vi "SECADO_JKI.vi"() -> ()   [LabVIEW 2017] (continued)
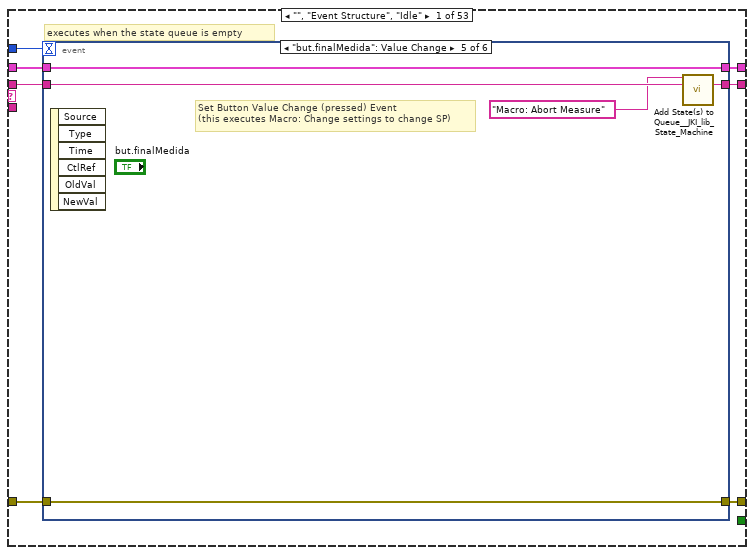
[diagram p2: hidden frame]
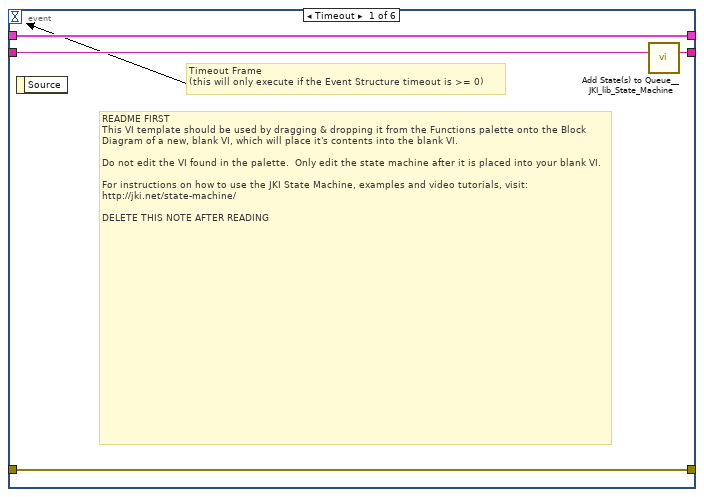
[diagram p3: hidden frame]
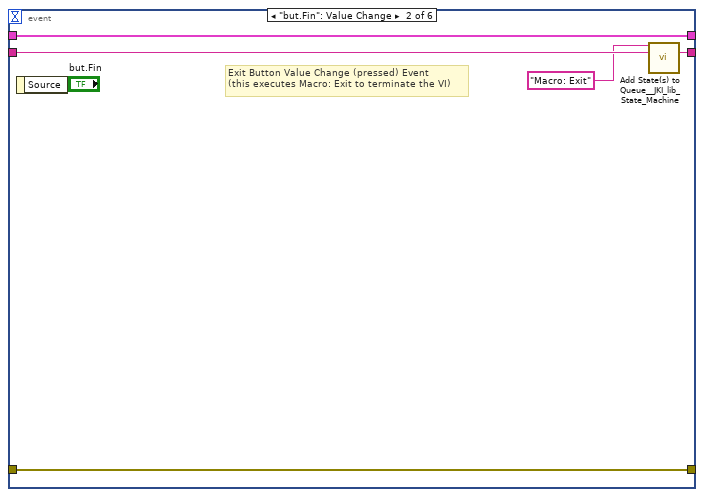
[diagram p4: hidden frame]
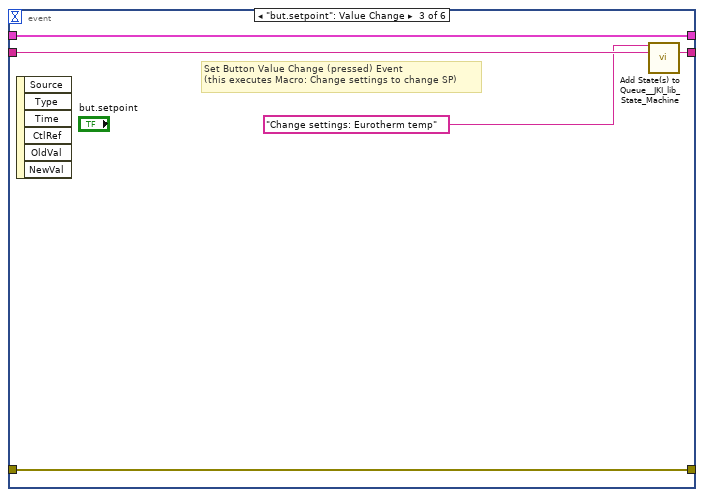
[diagram p5: hidden frame]
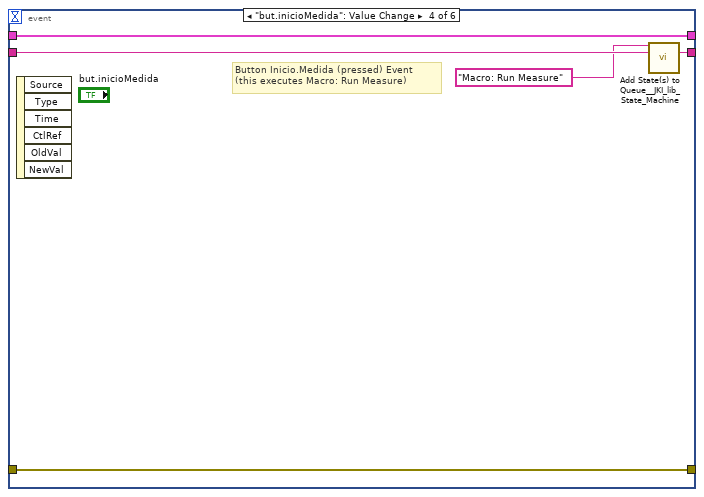
[diagram p6: hidden frame]
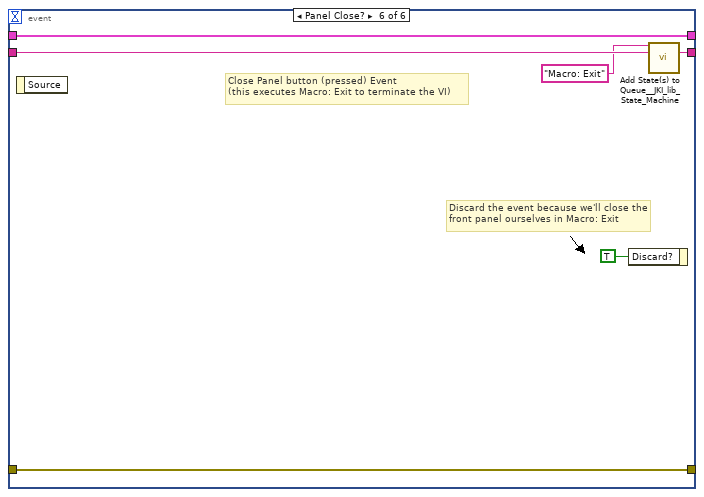
[diagram p7: hidden frame]
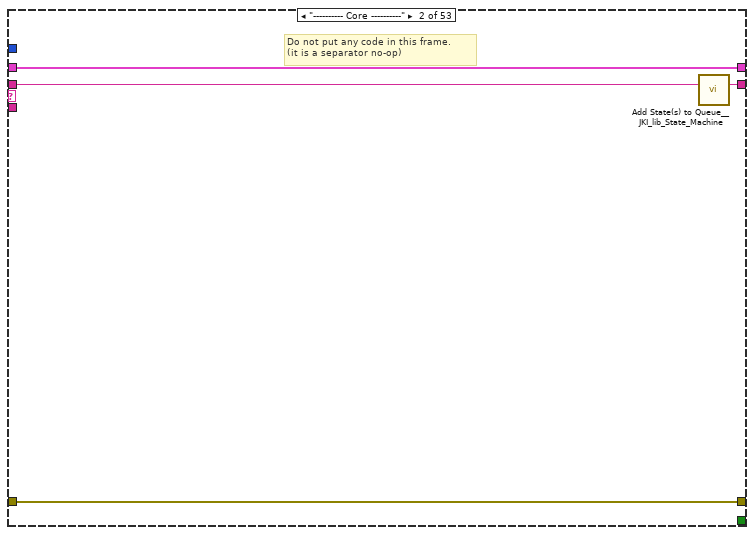
[diagram p8: hidden frame]
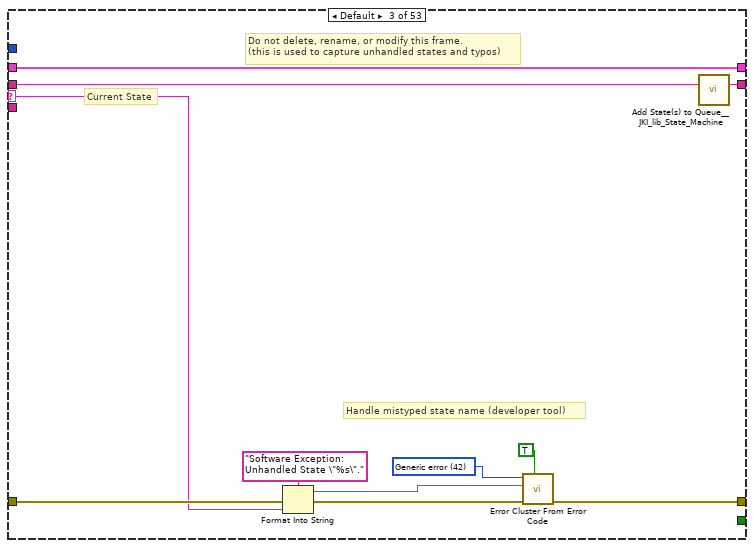
[diagram p9: hidden frame]
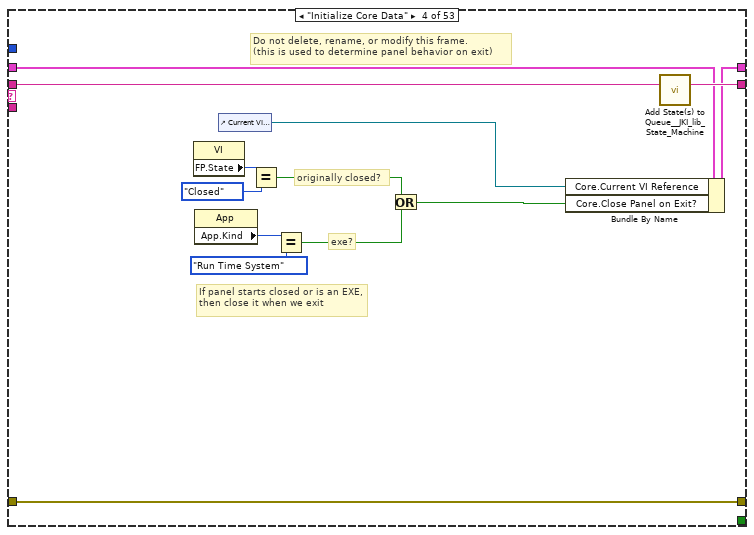
[diagram p10: hidden frame]
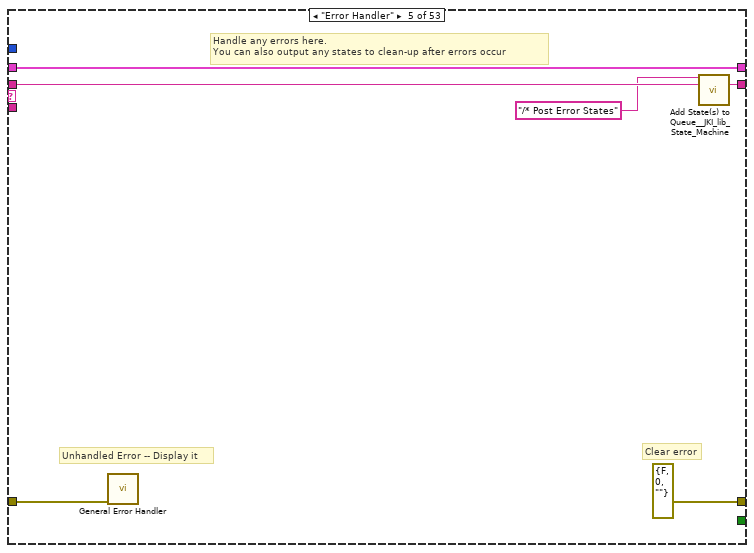
[diagram p11: hidden frame]
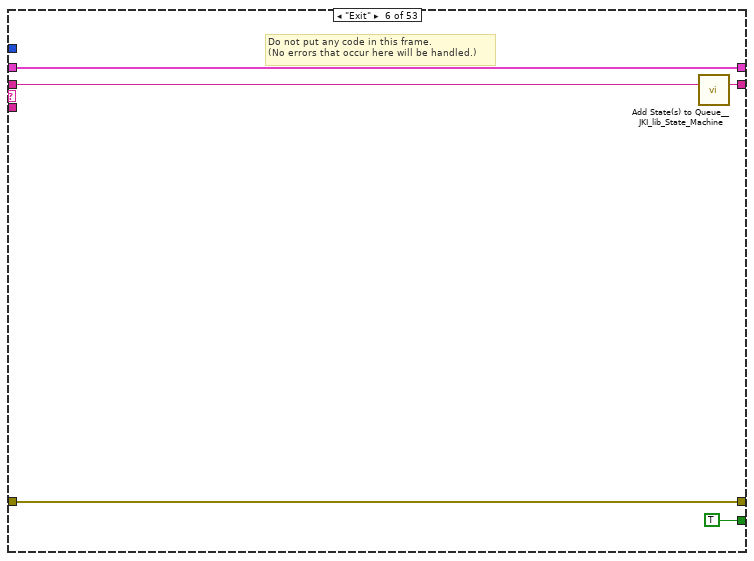
[diagram p12: hidden frame]
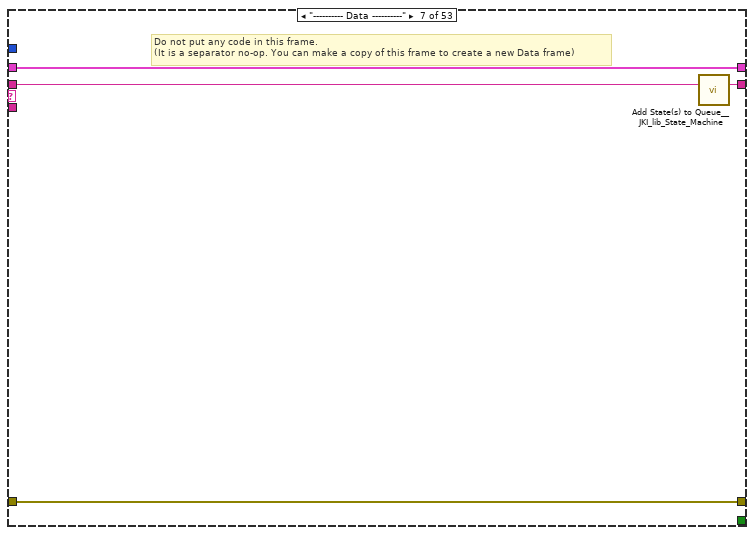
[diagram p13: hidden frame]
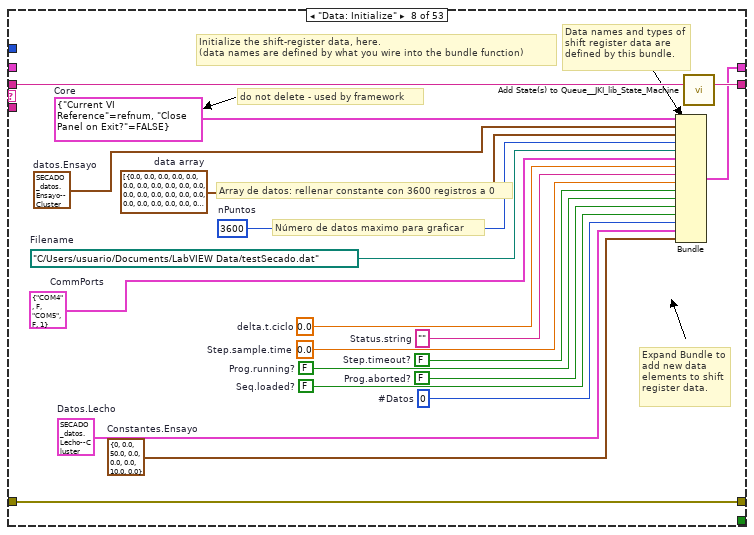
[diagram p14: hidden frame]
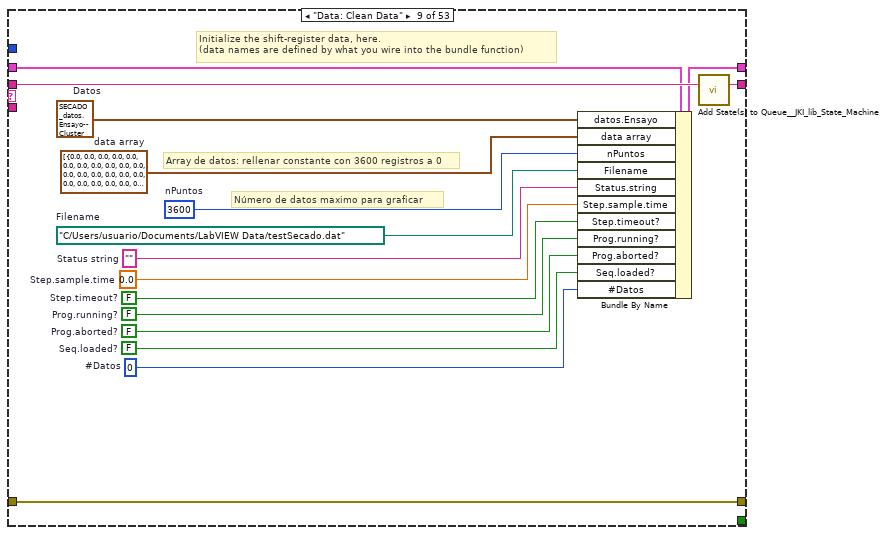
[diagram p15: hidden frame]
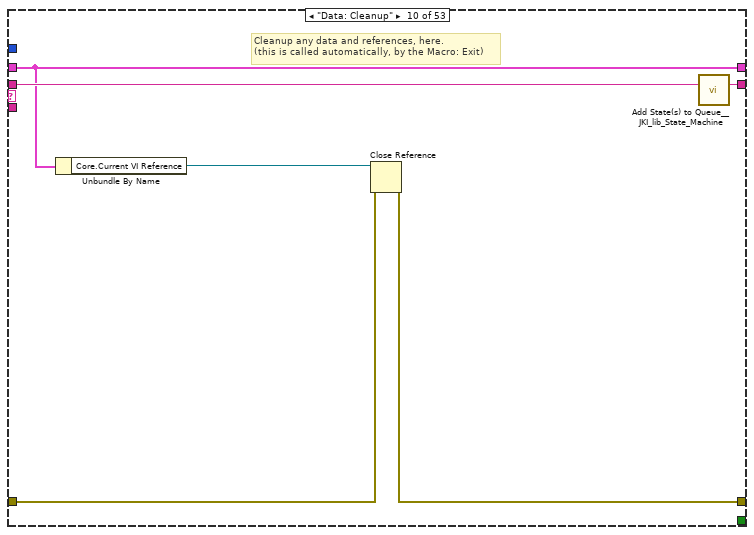
[diagram p16: hidden frame]
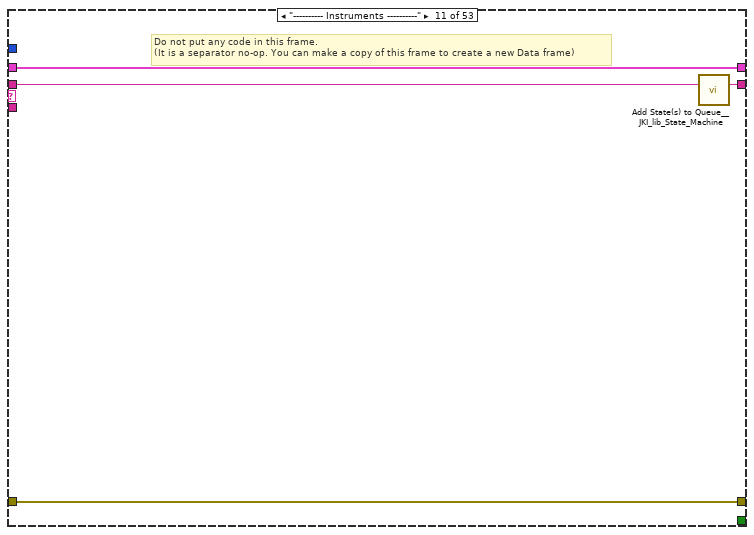
[diagram p17: hidden frame]
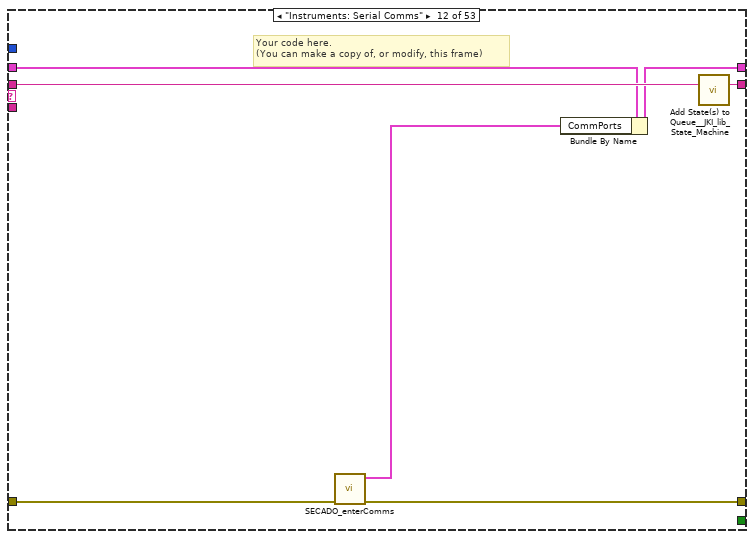
[diagram p18: hidden frame]
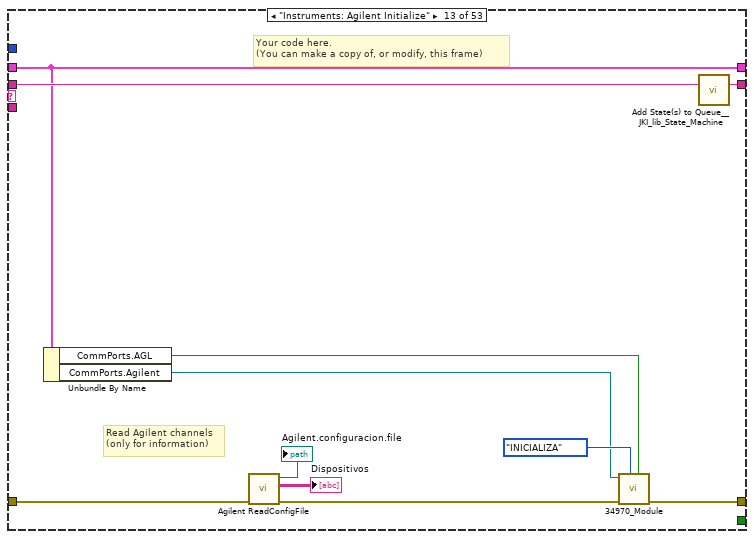
[diagram p19: hidden frame]
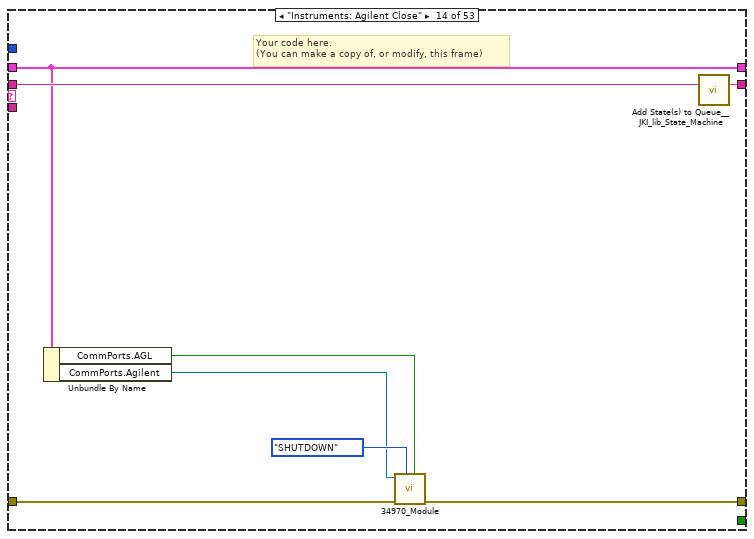
[diagram p20: hidden frame]
          tunnel: [w438] -> w406 mode=indexing
          tunnel: [w437] -> w407 mode=indexing
          tunnel: [w436] -> w408 mode=indexing
          tunnel: [w435] -> w409 mode=indexing
          tunnel: [w434] -> w410 mode=indexing
          tunnel: [w433] -> w399 mode=indexing
          tunnel: [w432] -> w400 mode=indexing
          tunnel: [w431] -> w401 mode=indexing
          tunnel: [w430] -> w402 mode=indexing
          tunnel: [w429] -> w403 mode=indexing
          tunnel: w396 -> [w428] mode=indexing
          tunnel: [w427] -> w371 mode=indexing
          tunnel: [w426] -> w370 mode=indexing
          tunnel: [w425] -> w369 mode=indexing
          tunnel: [w424] -> w368 mode=indexing
          tunnel: [w423] -> w367 mode=indexing
          tunnel: [w422] -> w366 mode=indexing
          tunnel: [w421] -> w365 mode=indexing
          tunnel: [w420] -> w364 mode=indexing
          tunnel: [w419] -> w363 mode=indexing
          tunnel: [w418] -> w351 mode=indexing
          n120 = Unbundle By Name(w428) -> ("Tiempo (min)"=w441:dbl, "P116.set.temp, C"=w440:dbl, "P116.temperatura, C"=w439:dbl, "Temp.pt100.1, C"=w438:dbl, "Temp.pt100.2, C"=w437:dbl, "Q.set.caudal, g/s"=w436:dbl, "Q.caudal, g/s"=w435:dbl, "P116.output, W"=w434:dbl, "Humedad.lecho, f1"=w433:dbl, "Agua.evapor, g/s"=w432:dbl, "Q.aire.seco, W"=w431:dbl, "Q.evaporacion, W"=w430:dbl, "Temperatura.ext, C"=w429:dbl, "Temp.pt100.3, C"=w427:dbl, "Temp.pt100.4, C"=w426:dbl, "Temp.termopar.5, C"=w425:dbl, "Temp.termopar.6, C"=w424:dbl, "Humedad.rel.3, f1"=w423:dbl, "Humedad.rel.4, f1"=w422:dbl, "Presion.dif, Pa"=w421:dbl, "Vel.arrastre, m/s"=w420:dbl, "Vel.arrastre, m/s"=w419:dbl, "Vel.arrastre, m/s"=w418:dbl)
        }
        n121 = Bundle(w352, w404) -> (w394:cluster{dbl[], dbl[]})  [unwired: 1 in]
        n122 = Bundle(w352, w405) -> (w393:cluster{dbl[], dbl[]})  [unwired: 1 in]
        n123 = Bundle(w352, w406) -> (w392:cluster{dbl[], dbl[]})  [unwired: 1 in]
        n124 = Bundle(w352, w407) -> (w391:cluster{dbl[], dbl[]})  [unwired: 1 in]
        n125 = Bundle(w352, w408) -> (w390:cluster{dbl[], dbl[]})  [unwired: 1 in]
        n126 = Bundle(w352, w409) -> (w389:cluster{dbl[], dbl[]})  [unwired: 1 in]
        n127 = Bundle(w352, w410) -> (w388:cluster{dbl[], dbl[]})  [unwired: 1 in]
        n128 = Bundle(w352, w399) -> (w387:cluster{dbl[], dbl[]})  [unwired: 1 in]
        n129 = Bundle(w352, w400) -> (w386:cluster{dbl[], dbl[]})  [unwired: 1 in]
        n130 = Bundle(w352, w401) -> (w385:cluster{dbl[], dbl[]})  [unwired: 1 in]
        n131 = Bundle(w352, w402) -> (w384:cluster{dbl[], dbl[]})  [unwired: 1 in]
        n132 = Bundle(w352, w403) -> (w377:cluster{dbl[], dbl[]})  [unwired: 1 in]
        n133 = Bundle(w352, w371) -> (w362:cluster{dbl[], dbl[]})  [unwired: 1 in]
        n134 = Bundle(w352, w370) -> (w361:cluster{dbl[], dbl[]})  [unwired: 1 in]
        n135 = Bundle(w352, w369) -> (w360:cluster{dbl[], dbl[]})  [unwired: 1 in]
        n136 = Bundle(w352, w368) -> (w359:cluster{dbl[], dbl[]})  [unwired: 1 in]
        n137 = Bundle(w352, w367) -> (w358:cluster{dbl[], dbl[]})  [unwired: 1 in]
        n138 = Bundle(w352, w366) -> (w357:cluster{dbl[], dbl[]})  [unwired: 1 in]
        n139 = Bundle(w352, w365) -> (w356:cluster{dbl[], dbl[]})  [unwired: 1 in]
        n140 = Bundle(w352, w364) -> (w355:cluster{dbl[], dbl[]})  [unwired: 1 in]
        n141 = Bundle(w352, w363) -> (w354:cluster{dbl[], dbl[]})  [unwired: 1 in]
        n142 = Bundle(w352, w351) -> (w353:cluster{dbl[], dbl[]})  [unwired: 1 in]
        n143 = Build Array(w387) -> (→"CONCENTRACION HUMEDAD":cluster{dbl[], dbl[]}[])
        n144 = Build Array(w386) -> (→"AGUA EVAPORADA AL AIRE":cluster{dbl[], dbl[]}[])
        n145 = Build Array(w394, w393, w392, w391) -> (→"EUROTHERM":cluster{dbl[], dbl[]}[])
        n146 = Build Array(w390, w389) -> (→"CAUDAL":cluster{dbl[], dbl[]}[])
        n147 = Build Array(w388) -> (→"POTENCIA CALEFACCION":cluster{dbl[], dbl[]}[])
        n148 = Build Array(w385, w384) -> (→"Q CEDIDO Y ABSORBIDO":cluster{dbl[], dbl[]}[])
        n149 = Build Array(w358, w357) -> (→"HUMEDAD":cluster{dbl[], dbl[]}[])
        n150 = Build Array(w356) -> (→"PRES_DIF":cluster{dbl[], dbl[]}[])
        n151 = Build Array(w377, w362, w361, w360, w359) -> (→"TEMPERATURA":cluster{dbl[], dbl[]}[])
        n152 = Build Array(w355, w354, w353) -> (→"VELOCIDADES":cluster{dbl[], dbl[]}[])
        n153 = Bundle By Name(cluster=w415, "data array"=w396) -> (w397:T18)
        n154 = call <vilib>:"Add State(s) to Queue__JKI_lib_State_Machine.vi"("State(s) in (\"\")"=w417) -> ("States Out"=w416:string)  [unwired: 14 in]
      }
      frame "---------- Macro ----------" {
        # "Do not put any code in this frame.\n(It is a separator no-op. You can make a copy of this frame to create a new Macro frame)"
        n155 = call <vilib>:"Add State(s) to Queue__JKI_lib_State_Machine.vi"("State(s) in (\"\")"=w445) -> ("States Out"=w444:string)  [unwired: 14 in]
      }
      frame "Macro: Inicializar" {
        w452 = "Data: Initialize\nData: Clean Data\nInitialize Core Data\nUI: Initialize\nUI: Front Panel State >> Open\nMacro: Interlock\nUI: Update Meas Data\nUI: Update Graphics\nInstruments: Serial Comms\nInstruments: Agilent Initialize\nInstruments: Eurotherm Initialize"  # Data: Initialize Data: Clean Data Initialize Core Data UI: Initialize UI: Front Panel State >> Open Macro: Interlock UI: Update Meas Data UI: Update Graphics Instruments: Serial Comms Instruments: Agilent Initialize Instruments: Eurotherm Initialize
        # "Initialization Macro\n(This is called once, when the VI starts)"
        n156 = Bundle By Name(cluster=w447, "Prog.running?"=TRUE ("Prog. Running?"), "Prog.aborted?"=FALSE ("Prog. Aborted?"), "Seq.loaded?"=FALSE ("Seq. Loaded?"), "Status.string"="Ready to start...") -> (w446:T18)
        n157 = call <vilib>:"Add State(s) to Queue__JKI_lib_State_Machine.vi"("State(s) in Front (\"\")"=w452, "State(s) in (\"\")"=w455) -> ("States Out"=w454:string)  [unwired: 13 in]
      }
      frame "Macro: Run Measure" {
        # "Run Measure Macro\n(This is called once, when the VI starts)"
        n158 = Bundle By Name(cluster=w462, "Prog.running?"=TRUE ("Prog. Running?"), "Prog.aborted?"=FALSE ("Prog. Aborted?"), "Seq.loaded?"=FALSE ("Seq. Loaded?"), "Status.string"="Adquisition in progress...") -> (w460:T18)
        n159 = call <vilib>:"Add State(s) to Queue__JKI_lib_State_Machine.vi"("State(s) in Front (\"\")"="UI: Initialize\nMacro: Interlock\nFile: Filename\nTiming: Initialize Total Time\nTiming: Initialize Sample Time\nMacro: Next Meas Cycle", "State(s) in (\"\")"=w465) -> ("States Out"=w464:string)  [unwired: 13 in]
      }
      frame "Macro: Abort Measure" {
        # "Abort Measure Macro\n(This is called when abort buton is pressed)"
        n160 = Bundle By Name(cluster=w470, "Prog.running?"=FALSE ("Prog. Running?"), "Prog.aborted?"=TRUE ("Prog. Aborted?"), "Seq.loaded?"=FALSE ("Seq. Loaded?"), "Status.string"="Adquisition aborted...") -> (w469:T18)
        n161 = One Button Dialog(message="Measure aborted") -> ()  [unwired: 1 in, 1 out]
        n162 = call <vilib>:"Add State(s) to Queue__JKI_lib_State_Machine.vi"("State(s) in (\"\")"="// Data: Set Seq. Aborted Flag >> True\n// Macro: Interlock\n// IO: Dwell  // finish current step (remove to abort immediately)\n// Data: Set Running Step >> -1\n// UI: Update Table Selection\n// Data: Set Seq. Aborted Flag >> False\nMacro: Interlock") -> ("States Out"=w475:string)  [unwired: 14 in]
      }
      frame "Macro: Next Meas Cycle" {
        # "Initialization Macro\n(This is called once, when the VI starts)"
        n163 = Unbundle By Name(w479) -> ("#Datos"=w477:i32)
        n164 = Increment(x=w477) -> (x+1=w476:i32)
        "#.datos" <- w476
        n165 = Bundle By Name(cluster=w479, "#Datos"=w476) -> (w478:T18)
        n166 = call <vilib>:"Add State(s) to Queue__JKI_lib_State_Machine.vi"("State(s) in Front (\"\")"="Timing: Measure Total Time\nMacro: Take Data\nMacro: Calculate\nMacro: Interlock\nFile: Save Data\nUI: Update Meas Data\nUI: Update Graphics\nSampling: Check For Next Sample", "State(s) in (\"\")"=w483) -> ("States Out"=w482:string)  [unwired: 13 in]
      }
      frame "Macro: Take Data" {
        # "Initialization Macro\n(This is called once, when the VI starts)"
        n167 = call <vilib>:"Add State(s) to Queue__JKI_lib_State_Machine.vi"("State(s) in Front (\"\")"="Measure data: Agilent Temp.PT100\nMeasure data: Agilent Temp.TERMOPAR\nMeasure data: Agilent Pressure\nMeasure data: Agilent Humidity\nMeasure data: Eurotherm Temperature", "State(s) in (\"\")"=w488) -> ("States Out"=w487:string)  [unwired: 13 in]
      }
      frame "Macro: Calculate" {
        # "Initialization Macro\n(This is called once, when the VI starts)"
        n168 = call <vilib>:"Add State(s) to Queue__JKI_lib_State_Machine.vi"("State(s) in Front (\"\")"="Calculations: Calculos 1", "State(s) in (\"\")"=w493) -> ("States Out"=w492:string)  [unwired: 13 in]
      }
      frame "Macro: Interlock" {
        # "Initialization Macro\n(This is called once, when the VI starts)"
        n169 = call <vilib>:"Add State(s) to Queue__JKI_lib_State_Machine.vi"("State(s) in Front (\"\")"="UI: Update Status\nUI: Update Interlock", "State(s) in (\"\")"=w498) -> ("States Out"=w497:string)  [unwired: 13 in]
      }
      frame "Macro: Exit" {
        # "Exit Macro\n(This is called once, when the VI exits)"
        n170 = Unbundle By Name(w506) -> ("Core.Close Panel on Exit?"=w505:bool)
        n171 = One Button Dialog(message="Program stop") -> ()  [unwired: 1 in, 1 out]
        n172 = Select(t="UI: Front Panel State >> Close", s=w505, f="") -> (s? t:f=w502:string)
        n173 = call <vilib>:"Add State(s) to Queue__JKI_lib_State_Machine.vi"("State(s) in (\"\")"=w502, "State(s) at Back (\"\")"="Data: Cleanup\nExit") -> ("States Out"=w500:string)  [unwired: 13 in]
        n174 = call <vilib>:"Add State(s) to Queue__JKI_lib_State_Machine.vi"("State(s) in Front (\"\")"=w500, "State(s) in (\"\")"=w509) -> ("States Out"=w508:string)  [unwired: 13 in]
      }
      frame "---------- File ----------" {
        # "Template Separator\n(You can make a copy of, or modify, this frame)"
        n175 = call <vilib>:"Add State(s) to Queue__JKI_lib_State_Machine.vi"("State(s) in (\"\")"=w513) -> ("States Out"=w512:string)  [unwired: 14 in]
      }
      frame "File: Filename" {
        # "Al arrancar la medida:\nHumedad.lecho = Humedad_inicial"
        # "Initialize and save head data"
        # "Your code here.\n(You can make a copy of, or modify, this frame)"
        n176 = call "SECADO_enterEnsayo.vi"("error in (no error)"=w520) -> ("error out"=w522:errorcluster, "Datos.Lecho"=w515:T5, "Constantes.Ensayo"=w516:T6)  [unwired: 7 in, 1 out]
        "Constantes.Ensayo" <- w516
        "Datos.Lecho" <- w515
        n177 = Unbundle By Name(w515) -> ("Hum_ini, %"=w514:dbl)
        n178 = call "File_Module.vi"("Command"=File_Module_Control."Initialize", "error in (no error)"=w522, "Datos.Lecho"=w515, "Constantes.Ensayo"=w516) -> ("error out"=w519:errorcluster, "selected path"=w517:path)  [unwired: 6 in]
        "Fichero" <- w517
        n179 = Bundle By Name(cluster=w523, "Constantes.Ensayo"=w516, "Datos.Lecho"=w515, "Filename"=w517, "datos.Ensayo.Humedad.lecho, f1"=w514) -> (w518:T18)
        n180 = call <vilib>:"Add State(s) to Queue__JKI_lib_State_Machine.vi"("State(s) in (\"\")"=w525) -> ("States Out"=w524:string)  [unwired: 14 in]
      }
      frame "File: Save Data" {
        # "Your code here.\n(You can make a copy of, or modify, this frame)"
        n181 = Get Date/Time String() -> (date string=→"Fecha":string, time string=→"Hora":string)  [unwired: 3 in]
        n182 = Unbundle By Name(w528) -> ("datos.Ensayo"=w529:T4)
        n183 = call "File_Module.vi"("Command"=File_Module_Control."Save Data", "error in (no error)"=w531, "Datos.Ensayo"=w529) -> ("error out"=w530:errorcluster)  [unwired: 7 in, 1 out]
        n184 = call <vilib>:"Add State(s) to Queue__JKI_lib_State_Machine.vi"("State(s) in (\"\")"=w534) -> ("States Out"=w533:string)  [unwired: 14 in]
      }
      frame "---------- Sampling ----------" {
        # "Template Separator\n(You can make a copy of, or modify, this frame)"
        n185 = call <vilib>:"Add State(s) to Queue__JKI_lib_State_Machine.vi"("State(s) in (\"\")"=w538) -> ("States Out"=w537:string)  [unwired: 14 in]
      }
      frame "Sampling: Check For Next Sample" {
        # "Your code here.\n(You can make a copy of, or modify, this frame)"
        n186 = Unbundle By Name(w544) -> ("Step.timeout?"=w542:bool)
        n187 = Select(t="Timing: Initialize Sample Time\nMacro: Next Meas Cycle", s=w542, f="Idle  //Calls event structure\nTiming: Measure Sample Time\nSampling: Check For Next Sample // Come back here") -> (s? t:f=w540:string)
        n188 = call <vilib>:"Add State(s) to Queue__JKI_lib_State_Machine.vi"("State(s) in Front (\"\")"=w540, "State(s) in (\"\")"=w546) -> ("States Out"=w545:string)  [unwired: 13 in]
      }
      frame "---------- Measure data ----------" {
        # "Template Separator\n(You can make a copy of, or modify, this frame)"
        n189 = call <vilib>:"Add State(s) to Queue__JKI_lib_State_Machine.vi"("State(s) in (\"\")"=w550) -> ("States Out"=w549:string)  [unwired: 14 in]
      }
      frame "Measure data: Agilent Temp.PT100" {
        # "Agilent temperature readings code here.\n(You can make a copy of, or modify, this frame)"
        n190 = Unbundle By Name(w553) -> ("CommPorts.AGL"=w551:bool, "CommPorts.Agilent"=w552:refnum<visa-resource-name>)
        n191 = call "34970_Module.vi"("Agilent 34970A"=w551, "Command"=34970_Module_Control."LECTURA PT100", "error in (no error)"=w554, "VISA Agilent 34970A"=w552) -> ("error out"=w555:errorcluster, "TEMP.PT100"=w561:dbl[])  [unwired: 3 in, 3 out]
        n192 = Index Array(array=w561) -> (element #1=w559:dbl, element #2=w558:dbl, element #3=w557:dbl, element #4=w556:dbl)  [unwired: 4 in]
        n193 = Bundle By Name(cluster=w553, "datos.Ensayo.Temp.pt100.1, C"=w559, "datos.Ensayo.Temp.pt100.2, C"=w558, "datos.Ensayo.Temp.pt100.3, C"=w557, "datos.Ensayo.Temp.pt100.4, C"=w556) -> (w560:T18)
        n194 = call <vilib>:"Add State(s) to Queue__JKI_lib_State_Machine.vi"("State(s) in (\"\")"=w564) -> ("States Out"=w563:string)  [unwired: 14 in]
      }
      frame "Measure data: Agilent Temp.TERMOPAR" {
        # "Agilent temperature readings code here.\n(You can make a copy of, or modify, this frame)"
        n195 = Unbundle By Name(w567) -> ("CommPorts.AGL"=w565:bool, "CommPorts.Agilent"=w566:refnum<visa-resource-name>)
        n196 = call "34970_Module.vi"("Agilent 34970A"=w565, "Command"=34970_Module_Control."LECTURA TERMOPAR", "error in (no error)"=w568, "VISA Agilent 34970A"=w566) -> ("error out"=w569:errorcluster, "TEMP.PT100"=w574:dbl[])  [unwired: 3 in, 3 out]
        n197 = Index Array(array=w574) -> (element #1=w572:dbl, element #2=w571:dbl, element #3=w570:dbl)  [unwired: 3 in]
        n198 = Bundle By Name(cluster=w567, "datos.Ensayo.Temperatura.ext, C"=w572, "datos.Ensayo.Temp.termopar.5, C"=w571, "datos.Ensayo.Temp.termopar.6, C"=w570) -> (w573:T18)
        n199 = call <vilib>:"Add State(s) to Queue__JKI_lib_State_Machine.vi"("State(s) in (\"\")"=w577) -> ("States Out"=w576:string)  [unwired: 14 in]
      }
      frame "Measure data: Agilent Pressure" {
        # "Agilent pressure readings code here.\n(You can make a copy of, or modify, this frame)"
        n200 = Unbundle By Name(w582) -> ("CommPorts.AGL"=w580:bool, "CommPorts.Agilent"=w581:refnum<visa-resource-name>)
        n201 = call "34970_Module.vi"("Agilent 34970A"=w580, "Command"=34970_Module_Control."LECTURA PRESION", "error in (no error)"=w583, "VISA Agilent 34970A"=w581) -> ("error out"=w584:errorcluster, "PRESION"=w578:dbl[])  [unwired: 3 in, 3 out]
        n202 = Index Array(array=w578) -> (element=w585:dbl)  [unwired: 1 in]
        n203 = Bundle By Name(cluster=w582, "datos.Ensayo.Presion.dif, Pa"=w585) -> (w586:T18)
        n204 = call <vilib>:"Add State(s) to Queue__JKI_lib_State_Machine.vi"("State(s) in (\"\")"=w588) -> ("States Out"=w587:string)  [unwired: 14 in]
      }
      frame "Measure data: Agilent Humidity" {
        # "Agilent humidity readings code here.\n(You can make a copy of, or modify, this frame)"
        n205 = Unbundle By Name(w593) -> ("CommPorts.AGL"=w591:bool, "CommPorts.Agilent"=w592:refnum<visa-resource-name>)
        n206 = call "34970_Module.vi"("Agilent 34970A"=w591, "Command"=34970_Module_Control."LECTURA HUMEDAD", "error in (no error)"=w594, "VISA Agilent 34970A"=w592) -> ("error out"=w595:errorcluster, "HUMEDAD"=w589:dbl[])  [unwired: 3 in, 3 out]
        n207 = Index Array(array=w589) -> (element #1=w597:dbl, element #2=w596:dbl)  [unwired: 2 in]
        n208 = Bundle By Name(cluster=w593, "datos.Ensayo.Humedad.rel.3, f1"=w597, "datos.Ensayo.Humedad.rel.4, f1"=w596) -> (w598:T18)
        n209 = call <vilib>:"Add State(s) to Queue__JKI_lib_State_Machine.vi"("State(s) in (\"\")"=w600) -> ("States Out"=w599:string)  [unwired: 14 in]
      }
      frame "Measure data: Eurotherm Temperature" {
        # "POTENCIA MAXIMA"
        # "Your code here.\n(You can make a copy of, or modify, this frame)"
        n210 = Unbundle By Name(w624) -> ("CommPorts.CDT"=w618:bool, "CommPorts.Eurotherm"=w619:refnum<visa-resource-name>, "CommPorts.#Dec"=w604:u16)
        n211 = local read "Constantes.Ensayo"() -> (w603:T6)
        n212 = Unbundle By Name(w603) -> ("Voltaje_resist, vac"=w601:dbl, "Resistencia, ohm"=w602:dbl)
        n213 = call "Eurotherm_2023_Module.vi"("Eurotherm (T:Enable)"=w618, "Command"=Eurotherm_2023_Module."Initialize", "error in (no error)"=w623, "VISA resource name"=w619) -> ("error out"=w616:errorcluster)  [unwired: 5 in, 2 out]
        n214 = Square(x=w601) -> (x^2=w612:dbl)
        n215 = call "Eurotherm_2023_Module.vi"("Decimales"=w604, "Eurotherm (T:Enable)"=w618, "Command"=Eurotherm_2023_Module."Read data", "error in (no error)"=w616, "Address"=Address."Add 1", "VISA resource name"=w619) -> ("error out"=w615:errorcluster, "Eurotherm"=w614:T20)  [unwired: 3 in, 1 out]
        n216 = Divide(x=w612, y=w602) -> (x/y=w611:dbl)
        n217 = Unbundle By Name(w614) -> ("workingSP"=w608:dbl, "processVal"=w607:dbl, "workingOut"=w605:dbl)
        n218 = Multiply(x=w605, y=w611) -> (x*y=w610:dbl)
        n219 = Divide(x=w610, y=100.0) -> (x/y=w606:dbl)
        n220 = call "Eurotherm_2023_Module.vi"("Eurotherm (T:Enable)"=w618, "Command"=Eurotherm_2023_Module."Shutdown", "error in (no error)"=w615, "VISA resource name"=w619) -> ("error out"=w621:errorcluster)  [unwired: 5 in, 2 out]
        n221 = Bundle By Name(cluster=w624, "datos.Ensayo.P116.set.temp, C"=w608, "datos.Ensayo.P116.temperatura, C"=w607, "datos.Ensayo.P116.output, %"=w605, "datos.Ensayo.P116.output, W"=w606) -> (w620:T18)
        n222 = call <vilib>:"Add State(s) to Queue__JKI_lib_State_Machine.vi"("State(s) in (\"\")"=w627) -> ("States Out"=w626:string)  [unwired: 14 in]
      }
      frame "---------- Change settings ----------" {
        # "Template Separator\n(You can make a copy of, or modify, this frame)"
        n223 = call <vilib>:"Add State(s) to Queue__JKI_lib_State_Machine.vi"("State(s) in (\"\")"=w631) -> ("States Out"=w630:string)  [unwired: 14 in]
      }
      frame "Change settings: Eurotherm temp" {
        # "Your code here.\n(You can make a copy of, or modify, this frame)"
        n224 = Unbundle By Name(w641) -> ("datos.Ensayo.P116.set.temp, C"=w633:dbl, "CommPorts"=w638:T17, "CommPorts.CDT"=w640:bool, "CommPorts.Eurotherm"=w639:refnum<visa-resource-name>, "CommPorts.#Dec"=w637:u16)
        n225 = Bundle By Name(cluster=T15 {"TargetSP"={"Ch1"=0.0}, "WorkingSP"={"Ch1"=0.0}, "Temperatura"={"Ch1"=0.0}, "RateSP"={"Ch1"=0.0}, "Potencia"={"Ch1"=0.0}, "Potencia max"={"Ch1"=0.0}} ("P116x1ch"), "RateSP.Ch1"=0.0, "TargetSP.Ch1"=w633) -> (w635:T15)
        n226 = call "Eurotherm_2023_Module.vi"("Eurotherm (T:Enable)"=w640, "Command"=Eurotherm_2023_Module."Initialize", "error in (no error)"=w642, "VISA resource name"=w639) -> ("error out"=w646:errorcluster)  [unwired: 5 in, 2 out]
        n227 = call "P116x1ch_WriteManual.vi"("P116x1ch"=w635, "Decimales"=w637, "error in (no error)"=w646, "Comunicaciones"=w638) -> ("error out"=w645:errorcluster)  [unwired: 5 in, 2 out]
        n228 = call "Eurotherm_2023_Module.vi"("Eurotherm (T:Enable)"=w640, "Command"=Eurotherm_2023_Module."Shutdown", "error in (no error)"=w645, "VISA resource name"=w639) -> ("error out"=w636:errorcluster)  [unwired: 5 in, 2 out]
        n229 = call <vilib>:"Add State(s) to Queue__JKI_lib_State_Machine.vi"("State(s) in (\"\")"=w648) -> ("States Out"=w647:string)  [unwired: 14 in]
      }
      frame "---------- Calculations ----------" {
        # "Template Separator\n(You can make a copy of, or modify, this frame)"
        n230 = call <vilib>:"Add State(s) to Queue__JKI_lib_State_Machine.vi"("State(s) in (\"\")"=w652) -> ("States Out"=w651:string)  [unwired: 14 in]
      }
      frame "Calculations: Calculos 1" {
        w655 = T2 {"Agua.evap, g/s"=0.0, "Hum.lecho, %"=1.0, "Q.aire.seco, W"=50.0, "Q.evaporacion, W"=230.0, "Porosidad"=60.0, "Vel.a.lecho, m/s"=1.0, "Vel.min.fluido, m/s"=10.0, "Vel.arrastre, m/s"=5.0}  # Calculos.Ensayo
        # "Set Front Panel Open or Closed\n(Usage: \"UI: Front Panel State >> Open|Close\")"
        n231 = Unbundle By Name(w667) -> ("Datos.Lecho"=w664:T5, "Constantes.Ensayo"=w665:T6, "datos.Ensayo"=w666:T4)
        n232 = call "SECADO_calculos.vi"("error in (no error)"=w669, "datos.Ensayo.in"=w666, "Constantes.Ensayo"=w665, "Datos.Lecho"=w664) -> ("error out"=w668:errorcluster, "datos.Ensayo.out"=w654:T4)  [unwired: 6 in]
        n233 = Unbundle By Name(w654) -> ("Agua.evapor, g/s"=w656:dbl, "Humedad.lecho, f1"=w657:dbl, "Q.aire.seco, W"=w658:dbl, "Q.evaporacion, W"=w659:dbl, "Porosidad,"=w660:dbl, "Vel.a.lecho, m/s"=w661:dbl, "Vel.min.fluido, m/s"=w662:dbl, "Vel.arrastre, m/s"=w663:dbl)
        n234 = Bundle By Name(cluster=w655, "Agua.evap, g/s"=w656, "Hum.lecho, %"=w657, "Q.aire.seco, W"=w658, "Q.evaporacion, W"=w659, "Porosidad"=w660, "Vel.a.lecho, m/s"=w661, "Vel.min.fluido, m/s"=w662, "Vel.arrastre, m/s"=w663) -> (→"Calculos.Ensayo":T2)
        n235 = Bundle By Name(cluster=w667, "datos.Ensayo"=w654) -> (w670:T18)
        n236 = call <vilib>:"Add State(s) to Queue__JKI_lib_State_Machine.vi"("State(s) in (\"\")"=w672) -> ("States Out"=w671:string)  [unwired: 14 in]
      }
    }
    n237 = call <userlib>:"Wait (ms)__ogtk.vi"("error in (no error)"=w8, "milliseconds to wait"="t.wait, ms") -> ("error out"=w6:errorcluster)  [unwired: 8 in, 1 out]
    n238 = Unbundle By Name(w6) -> ("status"=→"Error":bool)
  }
  "error out" <- w2
  n239 = flat-sequence {
    tunnel: w2 -> [_]
    frame #0 {
      n240 = Quit LabVIEW(quit? (T)=TRUE) -> ()
    }
  }
